vi "Save Log File Module.vi"(7 "Log Header Parameters":T1={"Objective"=0, "Aline Rate"=2, "# Cscan"=1, "ROI Parameters"={"ROI (mm)"={"X (mm)"=1.0, "Y (mm)"=1.0}, "Shift (mm)"={"Xshift (mm)"=0.0, "Yshift (mm)"=0.0}}} {"Aline Rate" items=["76 KHz", "146 KHz", "76 KHz", "28 KHz", "10 KHz"]; "Objective" items=["5X LKM05", "10X LKM10", "20X LKM20", "10X LSM02"]}, 8 "error in (no error)":errorcluster, 9 "Scan Parameter":string="2048(Pix-Camera)-2048 (#Z Op)-0001(#Arpt)-05 (ArptExtra)-00400(#A)-060(BrtnExtra)-002(#Brpt)-400(#B)", 10 "Save Name":string="RAW-2048-0001-00400-002-400-", 11 "Save Path":path=path "E:/Jiarui/1217test") -> (0 "error out":errorcluster)   [LabVIEW 2017]
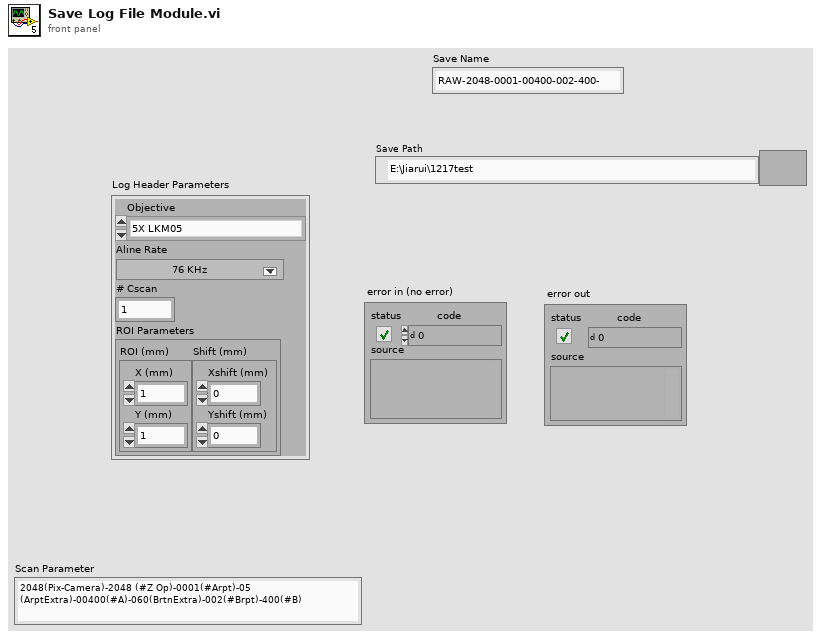
[diagram p1: front panel]
types:
  T1 = cluster{"Objective":u16, "Aline Rate":u16, "# Cscan":i32, "ROI Parameters":cluster{"ROI (mm)":cluster{"X (mm)":sgl, "Y (mm)":sgl}, "Shift (mm)":cluster{"Xshift (mm)":sgl, "Yshift (mm)":sgl}}}
  T2 = enum16{"open", "replace", "create", "open or create", "replace or create", "replace or create with confirmation"}
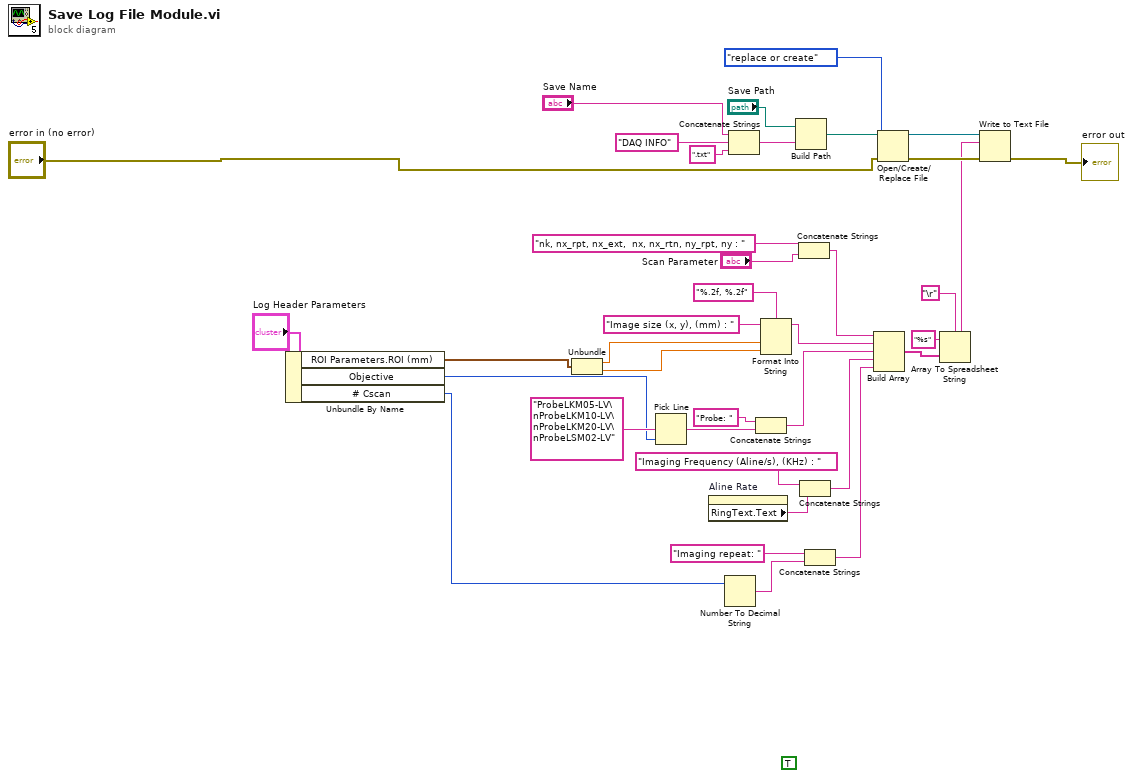
[diagram p0: block diagram]
diagram:
  (unwired) TRUE
  n1 = Unbundle By Name("Log Header Parameters") -> ("ROI Parameters.ROI (mm)"=w17:cluster{"X (mm)":sgl, "Y (mm)":sgl}, "Objective"=w14:u16, "# Cscan"=w9:i32)
  n2 = Unbundle(w17) -> ("X (mm)"=w16:sgl, "Y (mm)"=w15:sgl)
  n3 = Pick Line(multi-line string="ProbeLKM05-LV\nProbeLKM10-LV\nProbeLKM20-LV\nProbeLSM02-LV" ("string (\"\")"), line index=w14) -> (output string=w35:string)  [unwired: 1 in]
  n4 = property on="Aline Rate" class="Ring (strict)"() -> ("RingText.Text"=w11:string)  [unwired: 2 in, 2 out]
  n5 = Number To Decimal String(number=w9) -> (decimal integer string=w34:string)  [unwired: 1 in]
  n6 = Concatenate Strings("Save Name", "DAQ INFO" ("string"), ".txt" ("string")) -> (w29:string)
  n7 = Concatenate Strings("Probe: " ("string"), w35) -> (w13:string)
  n8 = Format Into String(format string="%.2f, %.2f", initial string="Image size (x, y), (mm) : " ("string"), w16, w15) -> (resulting string=w12:string)  [unwired: 1 in, 1 out]
  n9 = Build Path(base path="Save Path", name or relative path=w29) -> (appended path=w24:path)
  n10 = Concatenate Strings("nk, nx_rpt, nx_ext,  nx, nx_rtn, ny_rpt, ny : " ("string"), "Scan Parameter") -> (w2:string)
  n11 = Concatenate Strings("Imaging Frequency (Aline/s), (KHz) : " ("string"), w11) -> (w10:string)
  n12 = Concatenate Strings("Imaging repeat: " ("string"), w34) -> (w8:string)
  n13 = Build Array(w2, w12, w13, w10, w8) -> (w7:string[])
  n14 = Open/Create/Replace File(file path (use dialog)=w24, error in="error in (no error)", operation (0:open)=T2."replace or create") -> (refnum out=w22:refnum<file>, error out=w23:errorcluster)  [unwired: 3 in, 1 out]
  n15 = Array To Spreadsheet String(delimiter (Tab)="\r", array=w7, 3:"%s" ("format string")) -> (spreadsheet string=w6:string)
  n16 = Write to Text File(file (use dialog)=w22, text=w6, error in=w23) -> (error out=→"error out":errorcluster)  [unwired: 1 in, 2 out]
